vi "计算实际位置与理论位置在产品坐标系位置差异.vi"(10 "匹配后的实际影像坐标":cluster{dbl, dbl}[](array[cluster]), 11 "标准的影像坐标":cluster{dbl, dbl}[](array[cluster])) -> (3 "位置差异":cluster{dbl, dbl}[](array[cluster]))   [LabVIEW 2014]
uses:
  <vilib>/Analysis/coordinate.llb/2D Cartesian Coordinate Rotation (Scalar).vi
  <vilib>/Analysis/NI_AALPro.lvlib
panel:
  in  "Angle":dbl
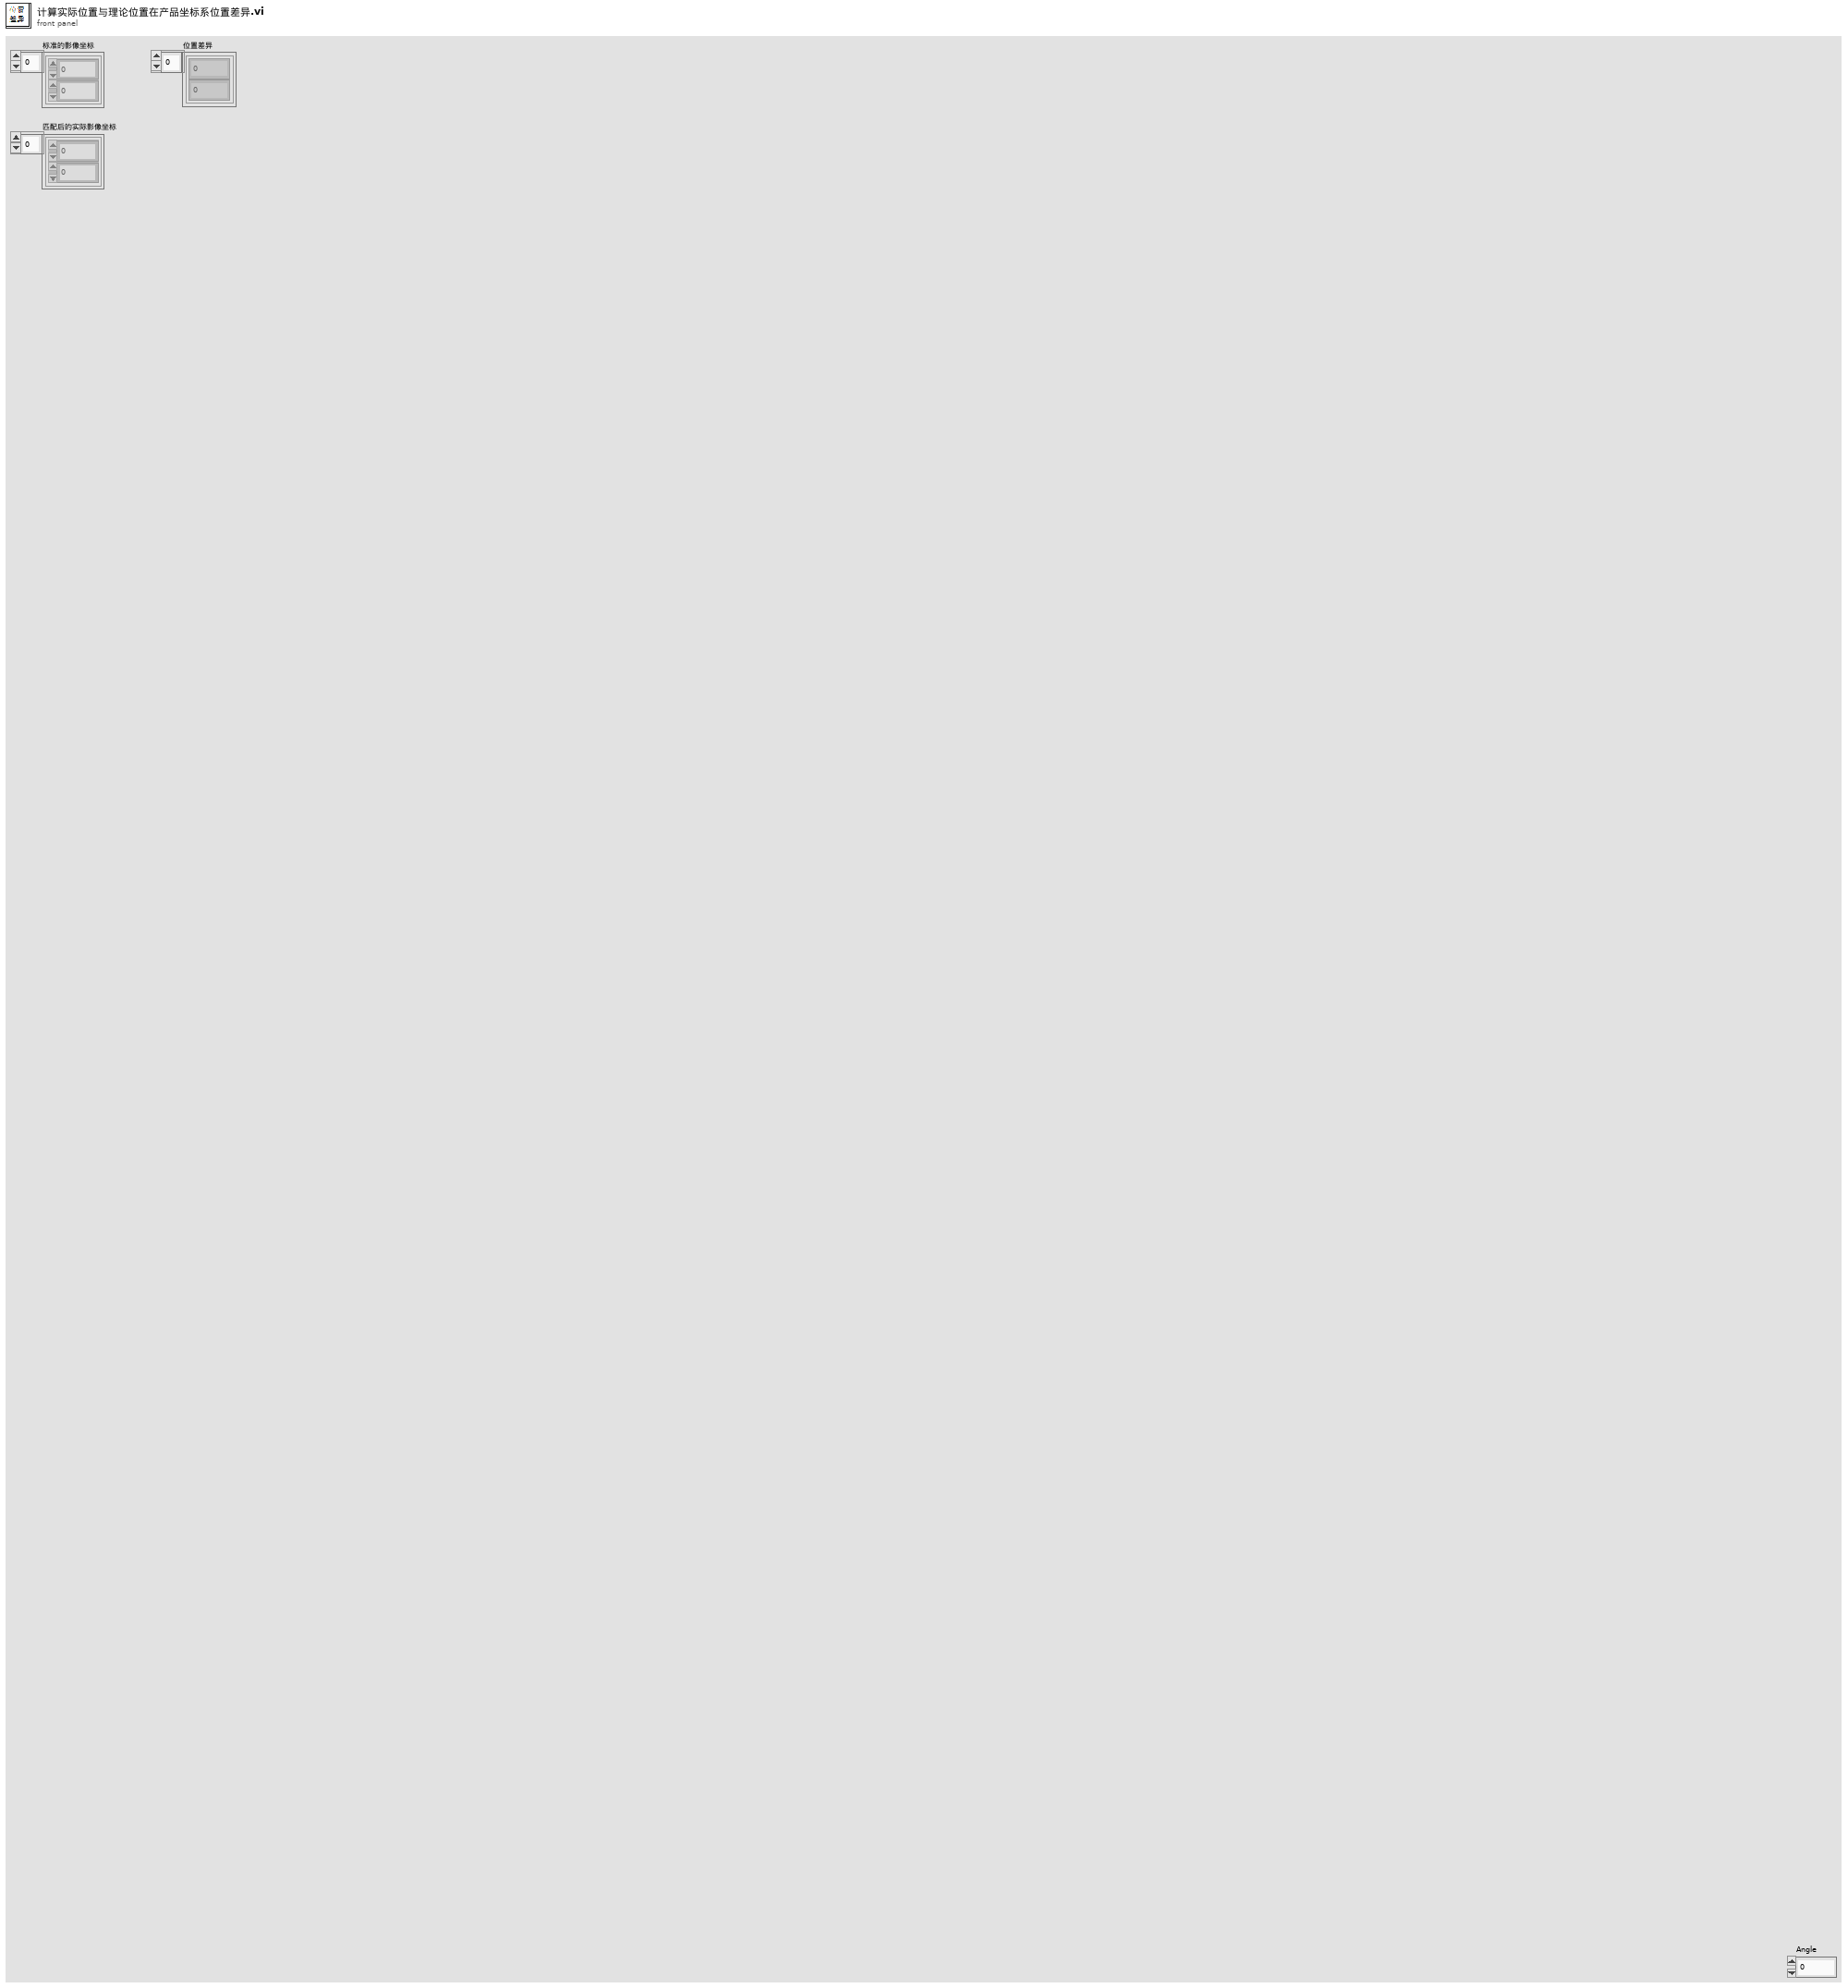
[diagram p1: front panel]
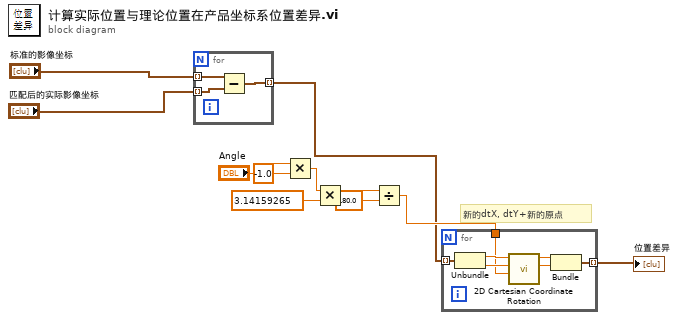
[diagram p0: block diagram]
diagram:
  # "新的dtX, dtY+新的原点"
  n1 = for {
    tunnel: "标准的影像坐标" -> [w14] mode=indexing
    tunnel: "匹配后的实际影像坐标" -> [w13] mode=indexing
    tunnel: [w12] -> w5 mode=indexing
    n2 = Subtract(x=w14, y=w13) -> (x-y=w12:cluster{dbl, dbl})
  }
  n3 = Multiply(x="Angle", y=-1.0) -> (x*y=w3:dbl)
  n4 = Multiply(x=w3, y=3.14159265) -> (x*y=w10:dbl)
  n5 = Divide(x=w10, y=180.0) -> (x/y=w8:dbl)
  n6 = for {
    tunnel: w8 -> [w15]
    tunnel: w5 -> [w21] mode=indexing
    tunnel: [w16] -> w1 mode=indexing
    n7 = Unbundle(w21) -> (w20:dbl, w19:dbl)
    n8 = call-poly <vilib>:"2D Cartesian Coordinate Rotation.vi"("theta"=w15, "y"=w19, "x"=w20) -> ("y out"=w17:dbl, "x out"=w18:dbl)  [unwired: 6 in, 1 out]
    n9 = Bundle("x out"=w18, "y out"=w17) -> (w16:cluster{"x out":dbl, "y out":dbl})  [unwired: 1 in]
  }
  "位置差异" <- w1
